vi "Get_IstanceName.vi"(8 "error in (no error)":errorcluster, 11 "ObserverClass in":refnum<class "ObserverClass.lvclass">) -> (0 "error out":errorcluster, 2 "IstanceName":string, 3 "ObserverClass out":refnum<class "ObserverClass.lvclass">)   [LabVIEW 2025, in "ObserverClass.lvlib" / "ObserverClass.lvclass"]
uses:
  ObserverClass.lvclass
  ObserverClass.lvclass/ObserverClass.ctl
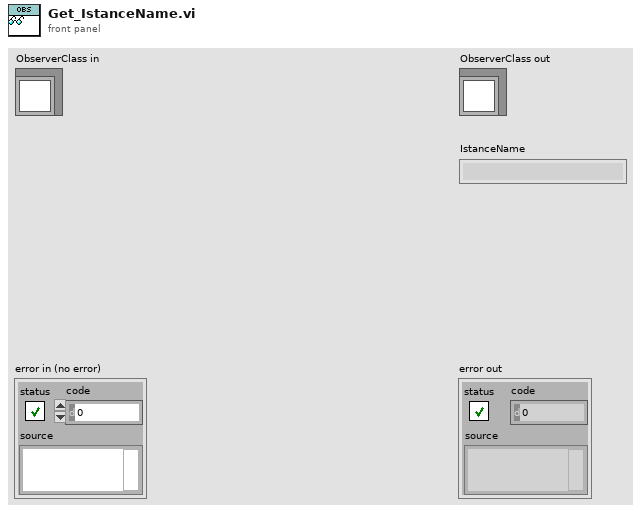
[diagram p1: front panel]
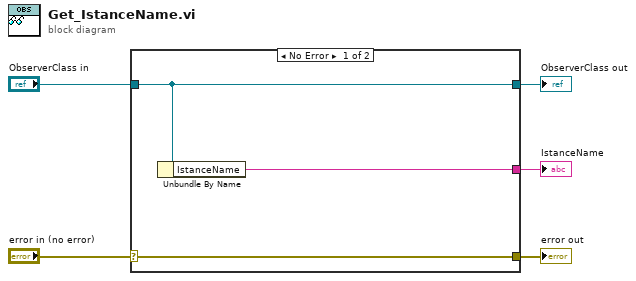
[diagram p0: block diagram]
diagram:
  n1 = case shown="No Error" "error in (no error)" {
    selector: "error in (no error)" -> [w8 w9]
    tunnel: [w8 w9] -> w4
    tunnel: [w7 w10] -> w2
    tunnel: "ObserverClass in" -> [w7 w10]
    tunnel: [w6 _] -> w1
    frame No Error {
      n2 = Unbundle By Name(w7) -> ("IstanceName"=w6:string)
    }
    frame Error {
    }
  }
  "error out" <- w4
  "ObserverClass out" <- w2
  "IstanceName" <- w1
